vi "Meas_Fast_FID_Bkgnd.vi"(3 "Mode":T6, 5 "Traverse line In":T3 {"Carrier_2 Q (l/min)" format="%#.2f"; "Row Duration (mins)" format="%#.1f"; "Row No" min=0; "Trace Gas Concentration (%)" min=0.0 format="%#_4f"; "Carrier_1 Q (l/min)" format="%#.4f"; "Start X" format="%#.2f"; "Start Y" format="%#.2f"; "Start Z" format="%#.2f"; "End X" format="%#.2f"; "End Y" format="%#.2f"; "End Z" format="%#.2f"; "Tunnel Speed" format="%#.2f"; "Averaging time (mins)" min=0.0 format="%#.2f"}) -> (0 "Error Message":string, 1 "Status":T2, 2 "Traverse line Out":T3 {"Carrier_2 Q (l/min)" format="%#.2f"; "Row Duration (mins)" format="%#.1f"; "Row No" min=0; "Trace Gas Concentration (%)" min=0.0 format="%#_4f"; "Carrier_1 Q (l/min)" format="%#.4f"; "Start X" format="%#.2f"; "Start Y" format="%#.2f"; "Start Z" format="%#.2f"; "End X" format="%#.2f"; "End Y" format="%#.2f"; "End Z" format="%#.2f"; "Tunnel Speed" format="%#.2f"; "Averaging time (mins)" min=0.0 format="%#.2f"})   [LabVIEW 2022 SP3]
uses:
  Gen Trav/Traverse_cluster.ctl
  Gen Trav/Spacing.ctl
  Controls/Multi_run_mode.ctl
  Controls/User_Specific_mode.ctl
  Gen Trav/Multi_Run_Status.ctl
  FFID/Bkgnd Meas.ctl
  File/Setup_Filetype.ctl
  Gen Trav/Trav_mode.ctl
  Controls/Setup.ctl
  Controls/Save_Data.ctl
  Globals/Trav_pos_global.vi
  Globals/Extra_Commands_Global.vi
  Globals/Preference_global.vi
  Globals/Gas_management_global.vi
  Globals/Meas_global.vi
  <vilib>/Analysis/NI_AALPro.lvlib
  <vilib>/Analysis/NI_AALBase.lvlib
panel:
  out "Bkgnd Results":T1[][](array[typedef])
  in  "Cluster":T1
  out "C^2 too large":bool
  out "Block Number":i32
  out "Can Move Traverse?":bool
  out "Trace Q":dbl
  out "Trace on?":bool
  out "After First Move":sgl[][](array[numeric])
  out "Traverses":string[](array[string])
  out "Initial Trav Positions":sgl[][](array[numeric])
  out "First Bknd since calib":bool
  # "X           Y          Z"
  # "Start"
  # "End"
  # "X           Y          Z"
  # "Start"
  # "End"
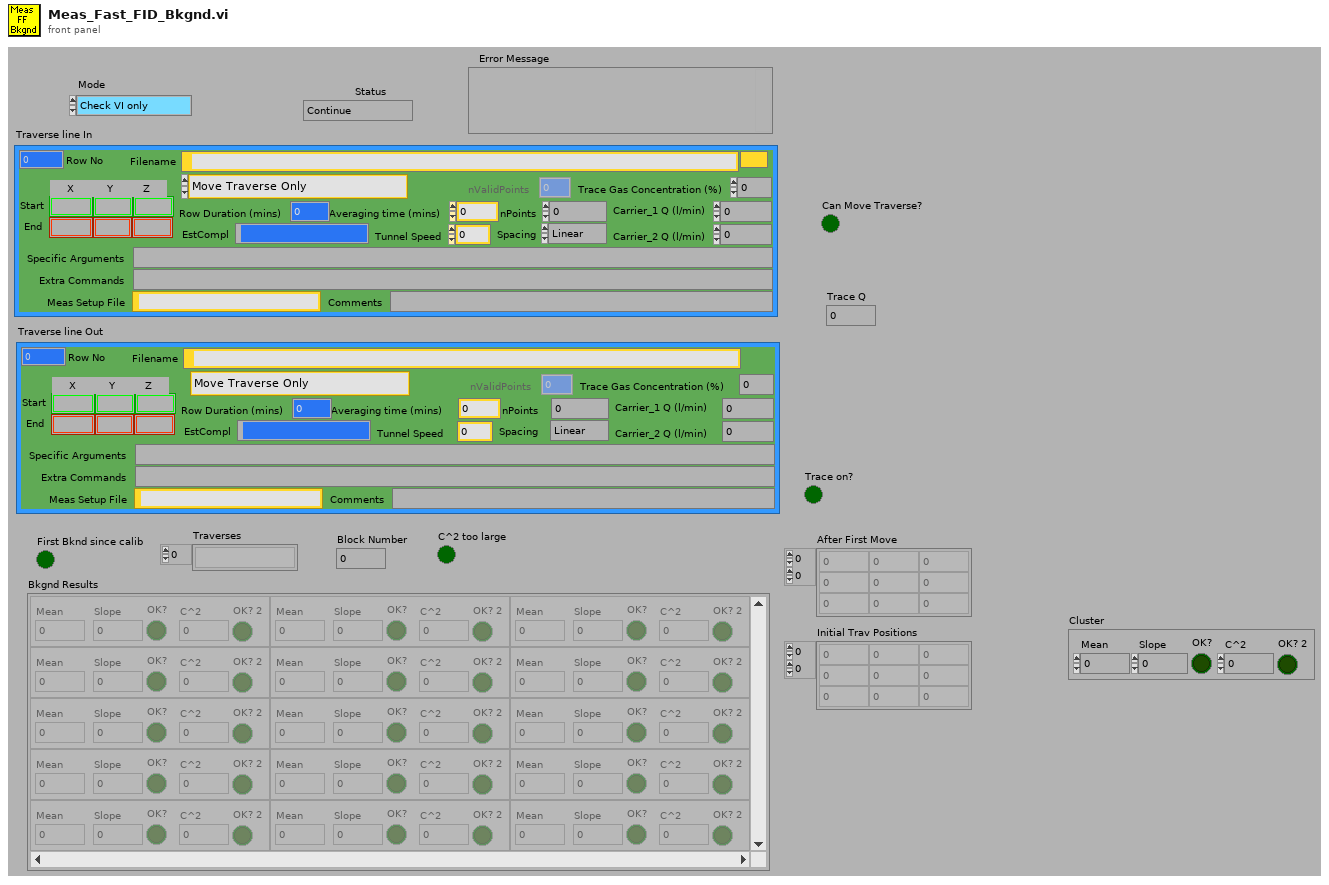
[diagram p1: front panel]
types:
  T1 = typedef "Bkgnd Meas.ctl" = cluster{"Mean":dbl, "Slope":dbl, "C^2":dbl, "OK?":bool, "OK? 2":bool}
  T2 = typedef "Multi_Run_Status.ctl" = enum16{"Continue", "Continue with Error", "Jump to Next Point", "Jump to Next Row", "Jump To Fall Back", "Terminate Run"}
  T3 = typedef "Traverse_cluster.ctl" = cluster{"Start X":sgl, "Start Y":sgl, "Start Z":sgl, "End X":sgl, "End Y":sgl, "End Z":sgl, "nPoints":i32, "Spacing":T4, "Filename":path, "Tunnel Speed":dbl, "Averaging time (mins)":dbl, "Extra Commands":string, "Carrier_1 Q (l/min)":dbl, "Carrier_2 Q (l/min)":dbl, "Trace Gas Concentration (%)":dbl, "Specific Arguments":string, "Comments":string, "Row No":i32, "Row Type Selector":T5, "EstCompl":string, "Row Duration (mins)":dbl, "nValidPoints":i32, "Meas Setup File":string}
  T4 = typedef "Spacing.ctl" = enum16{"Linear", "Log", "Gauss", "Specified", "N/A"}
  T5 = typedef "Multi_run_mode.ctl" = enum16{"Move Traverse Only", "Set Tunnel Speed Only", "Set Source Only", "Set Measurement Conditions", "Single Measurement", "Vertical Profile", "Lateral Profile", "Longitudinal Profile", "Multi-Axis Profile", "Explore Volume", "Auto Calibrate", "Meas Fast FID Bkgnd", "Check Beam Power", "Scanning Valve Measurement", "Run VI Named:", "Set ADAM Ch", "Wait (minutes)", "Send Message", "Synchronize With:", "Fall Back to this Row", "Turn Off Row Repeating", "Traverse 3D Volume", "Blank Row", "Jump to Fall Back Row"}
  T6 = typedef "User_Specific_mode.ctl" = enum16{"Check VI only", "Run VI"}
  T7 = typedef "Tunnel_Coordinates.ctl" = enum16{"Work in Tunnel Coordinates", "Work in Model Coordinates"}
  T8 = typedef "Setup_Filetype.ctl" = enum16{"Measurement Setups", "Calibration Setups", "General", "Results File Plotter Setups", "Speed Calib Tweaks"}
  T9 = typedef "Trav_mode.ctl" = enum16{"Move traverse", "Read traverse position", "Teach Position"}
  T10 = typedef "Save_Data.ctl" = enum16{"Save No Data", "Save Data"}
  T11 = typedef "Setup.ctl" = enum16{"Run Program", "Show Setup", "Save Current Setup", "Setup Front Panel"}
  T12 = typedef "GMU Gas Line Name.ctl" = enum16{"GMU1 Source", "GMU2 Source", "GMU2 Calib", "CPP GRC-A", "CPP GRC-B"}
  T13 = typedef "Analysis_info_cluster.ctl" = cluster{"Colour":u32, "Inst type":T14, "Inst name":string, "Symbol":string, "Code name":string, "Extra Info":string, "Inst Array":T15, "U":dbl, "u^2":dbl, "u^3":dbl, "u^4":dbl, "Skew_u":dbl, "Kurt_u":dbl, "Sd Error in Mean":dbl, "% u'/U":dbl, "X":dbl, "Y":dbl, "Z":dbl, "Timescale integral Estimate":dbl, "Sd Error in Variance":dbl, "Calib File":path, "Calib Constants":dbl[], "Output Position":bool, "Stats":enum16{"None", "Basic", "Full"}, "Av Sampling Rate":dbl, "Av No of Samples":dbl, "Total Meas Time (s)":dbl, "OrigChName":string, "Max value":dbl, "Min value":dbl, "Req Sample Rate Hz":dbl, "Sync Delay Time (s)":dbl, "Ch No":i16, "Device":string, "Use Latest Calib":bool, "Port":string, "Metadata Ch Names":string[], "Metadata Ch Values":string[], "Label":string, "chState":T16, "Point Drift":dbl, "inputConfig":string}
  T14 = typedef "Inst_type.ctl" = enum16{"Raw voltage", "Raw with zero offsetting", "Propeller anemometer", "Pressure Transducer", "Pitot-static tube", "Hot wire", "Cross wire 1", "Cross wire 2", "Generic Linear", "Generic Polynomial", "Generic BackPoly", "Fast FID", "Thermocouple", "Cold wire", "Pulsed Wire", "LDA Vel", "LDA Tran time", "LDA Arr time", "Microphone"}
  T15 = typedef "Instrument_Array.ctl" = enum16{"PWA", "LDA", "Analogue"}
  T16 = typedef "channelState.ctl" = enum32{"No Selection", "Solo", "Mute"}
  T17 = typedef "Time_Trace_Cluster.ctl" = cluster{"Weighting":dbl[], "Voltage":dbl[], "Eng Values":dbl[]}
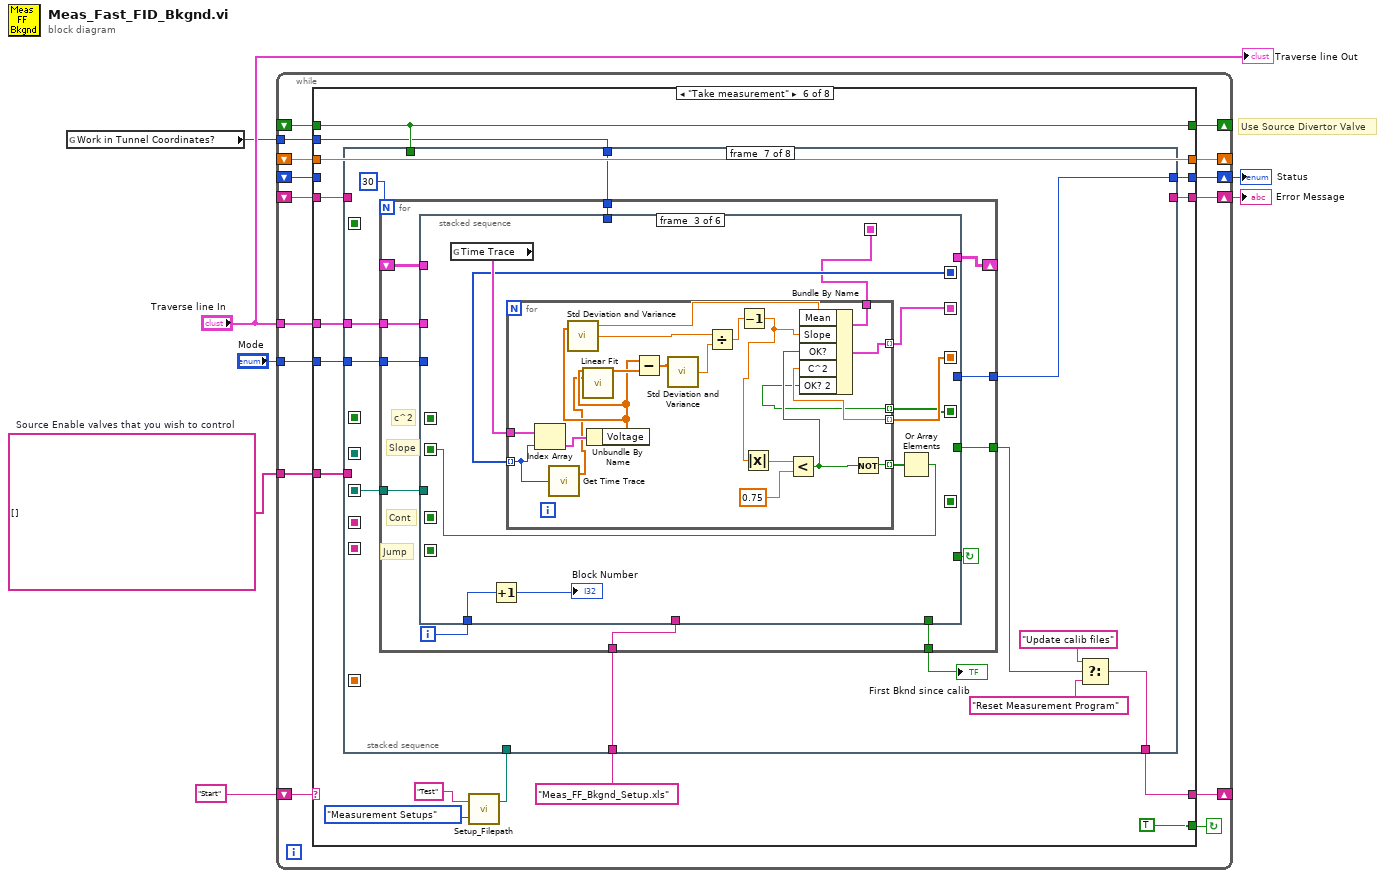
[diagram p0: block diagram]
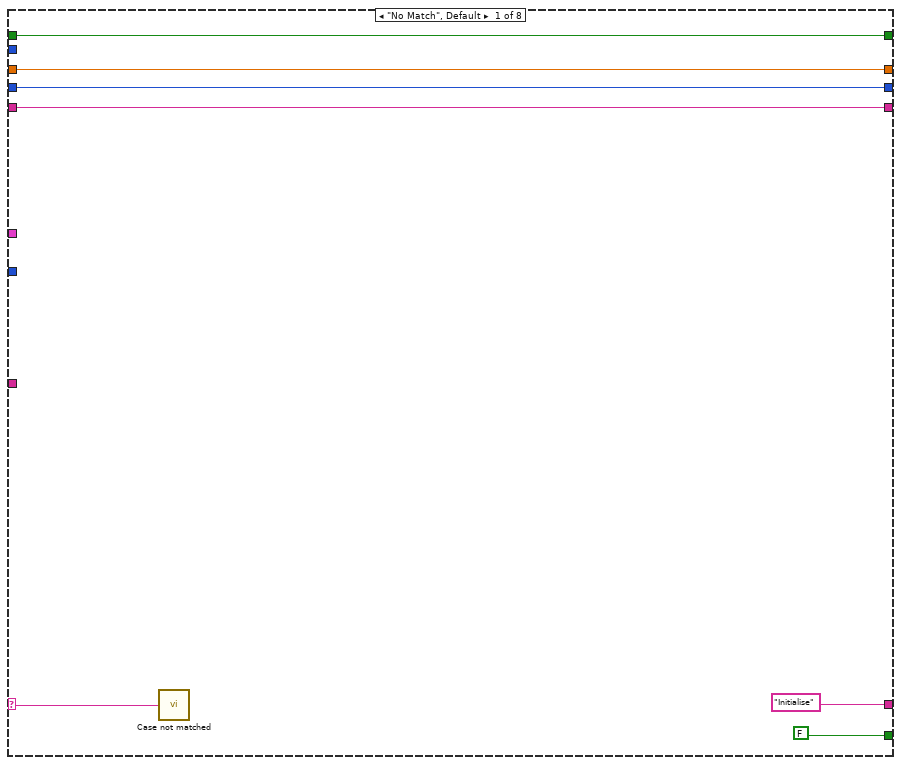
[diagram p2: hidden frame]
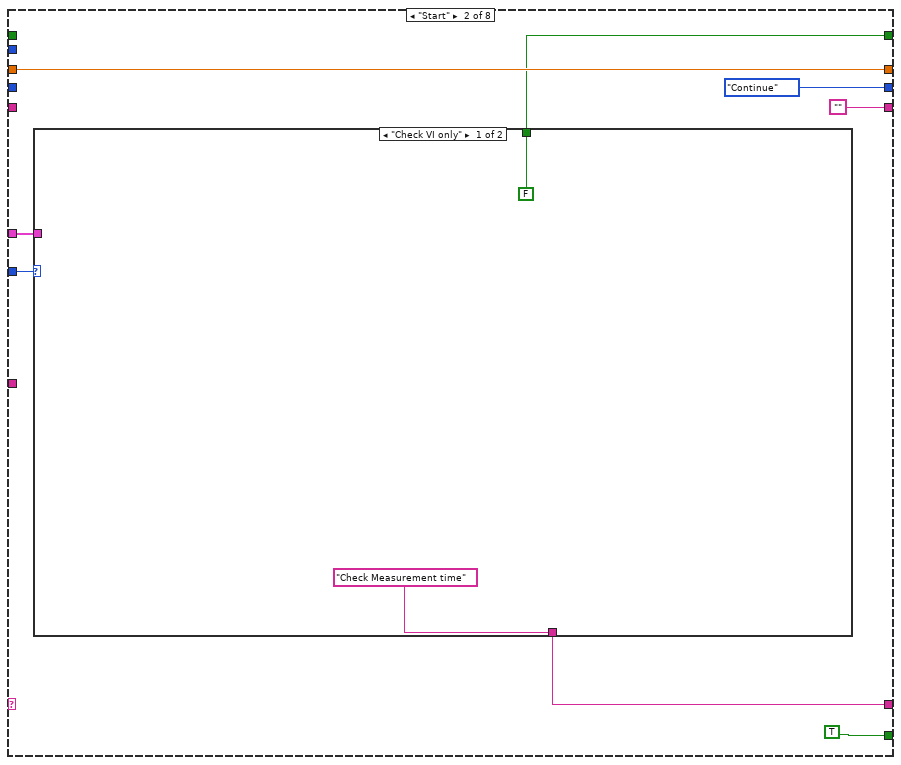
[diagram p3: hidden frame]
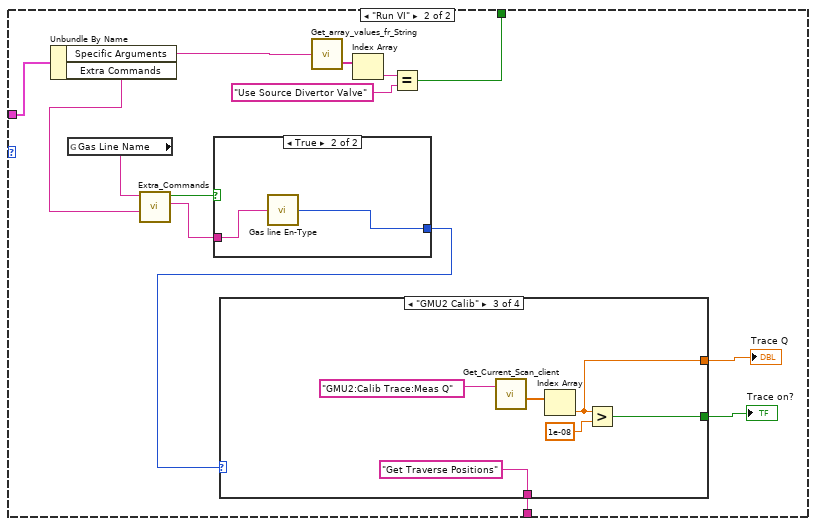
[diagram p4: hidden frame]
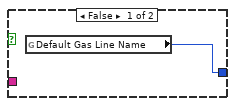
[diagram p5: hidden frame]
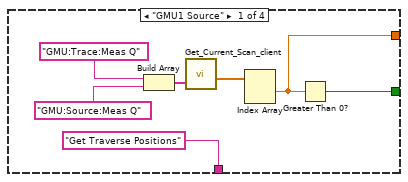
[diagram p6: hidden frame]
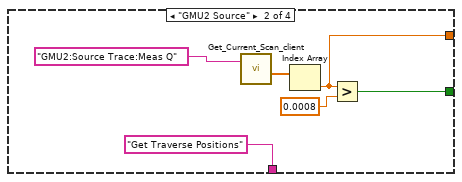
[diagram p7: hidden frame]
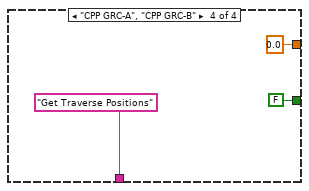
[diagram p8: hidden frame]
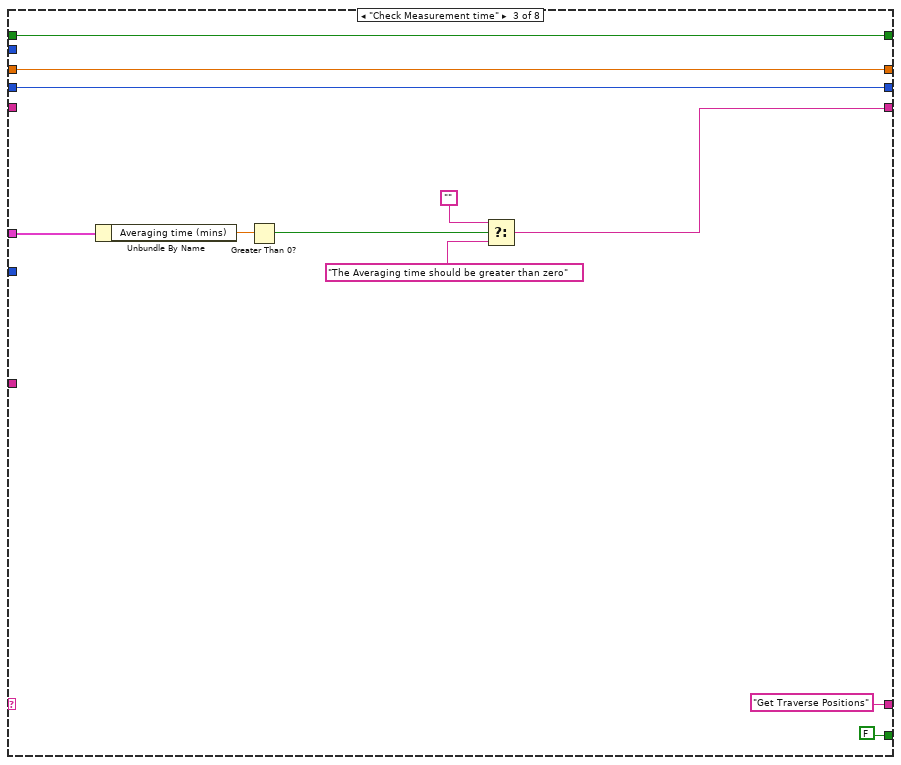
[diagram p9: hidden frame]
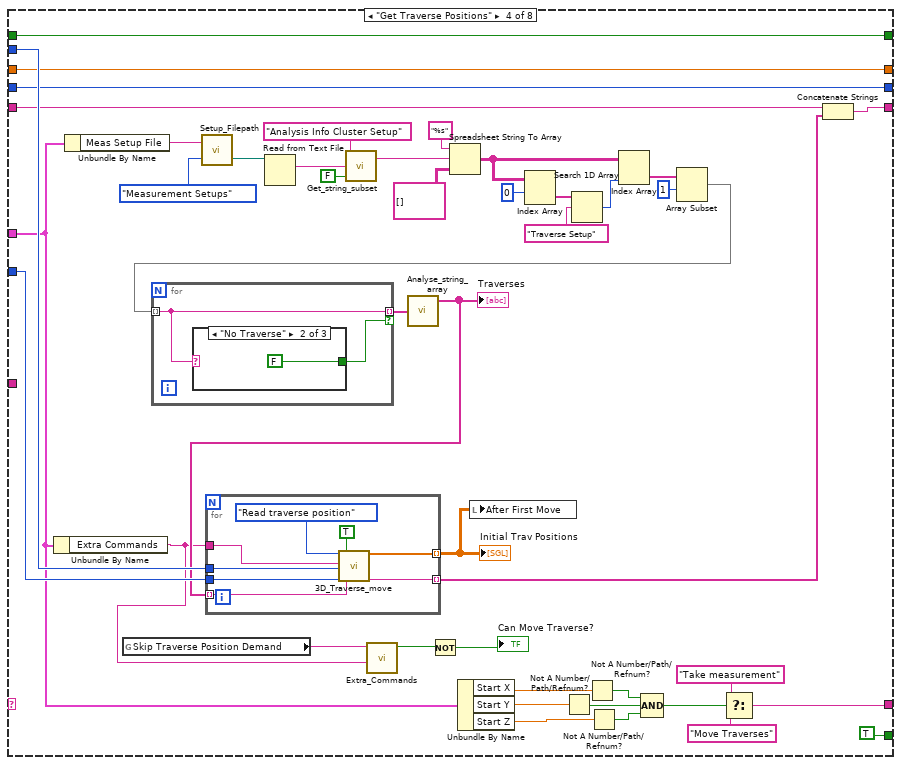
[diagram p10: hidden frame]
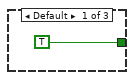
[diagram p11: hidden frame]
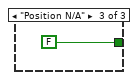
[diagram p12: hidden frame]
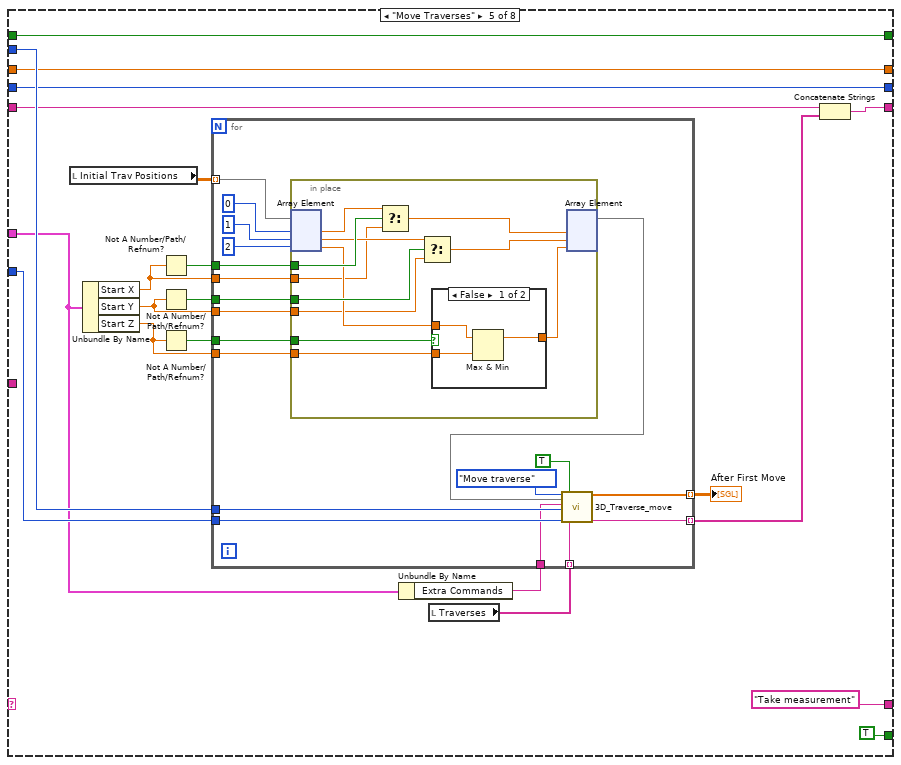
[diagram p13: hidden frame]
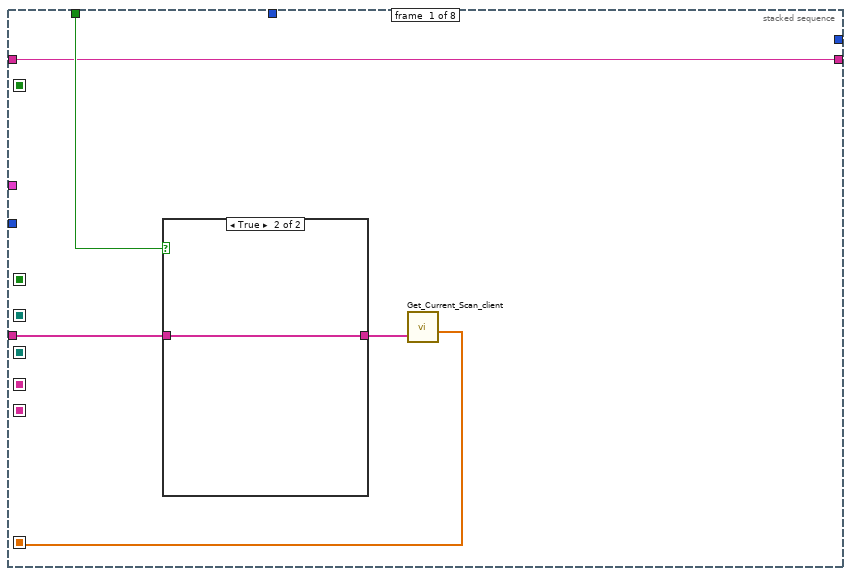
[diagram p15: hidden frame]
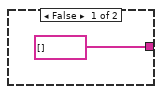
[diagram p16: hidden frame]
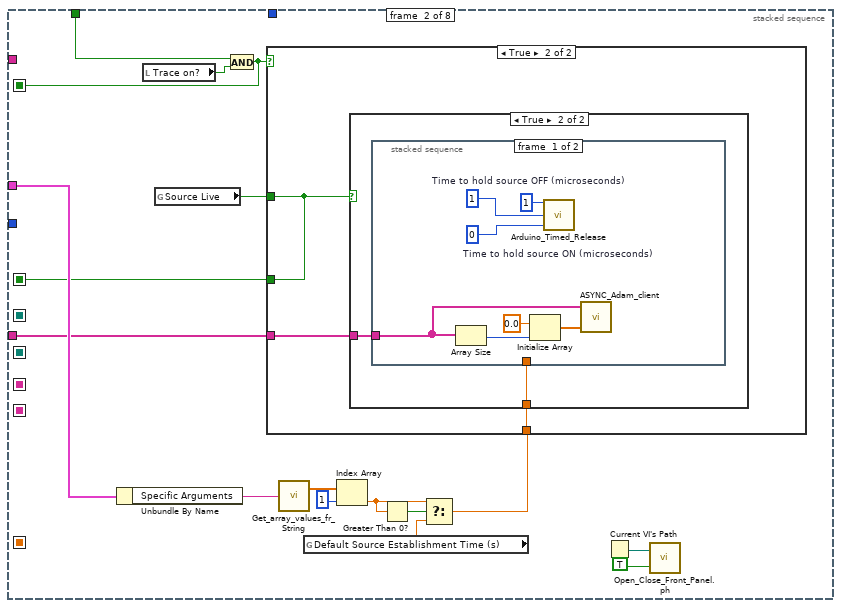
[diagram p17: hidden frame]
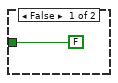
[diagram p18: hidden frame]
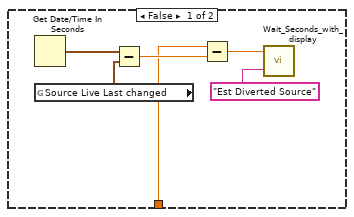
[diagram p19: hidden frame]
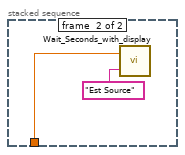
[diagram p20: hidden frame]
diagram:
  w1 = string[] []  # Source Enable valves that you wish to control
  # "Use Source Divertor Valve"
  n1 = global read "Trav_pos_global.vi" "Work in Tunnel Coordinates?"() -> (w2:T7)
  n2 = while {
    shift-left: "Start" -> [w20]
    shift-right: [w21] -> _
    shift-right: [w16] -> _
    shift-left: _ -> [w19]
    tunnel: "Mode" -> [w18]
    tunnel: "Traverse line In" -> [w17]
    shift-right: [w15] -> w5
    shift-left: _ -> [w13]
    shift-right: [w14] -> w3
    shift-left: _ -> [w12]
    tunnel: w2 -> [w11]
    shift-right: [w9] -> _
    shift-left: _ -> [w10]
    tunnel: w1 -> [w8]
    stop <- w22 continue-if-true
    n3 = case shown="\"Take measurement\"" w20 {
      selector: w20 -> [w23 _ _ _ _ _ _ _]
      tunnel: [FALSE TRUE FALSE TRUE TRUE TRUE TRUE FALSE] -> w22
      tunnel: ["Initialise" w35 "Get Traverse Positions" w120 "Take measurement" w212 "Reset Measurement Program" "End"] -> w21
      tunnel: w19 -> [w27 w33 w81 w127 w151 w216 w507 _]
      tunnel: w18 -> [_ w36 _ w129 w157 w207 _ _]
      tunnel: w17 -> [_ w30 w89 w95 w147 w215 _ _]
      tunnel: [w27 w33 w81 w127 w151 w216 w507 w512] -> w16
      tunnel: [w26 Multi_Run_Status."Continue" ("Status") w82 w126 w152 w213 w506 w511] -> w15
      tunnel: [w25 "" w85 w123 w154 w203 w505 w514] -> w14
      tunnel: w13 -> [w26 _ w82 w126 w152 _ w506 w511]
      tunnel: w12 -> [w25 _ _ w125 w155 w204 w505 w514]
      tunnel: w11 -> [_ _ _ w128 w156 w206 _ _]
      tunnel: w10 -> [w24 _ w80 w119 w167 w208 w502 w510]
      tunnel: [w24 w31 w80 w119 w167 w208 w502 w510] -> w9
      tunnel: w8 -> [_ _ _ _ _ w205 _ _]
      frame "No Match", Default {
        n4 = call "Case not matched.vi"("Case Name not Matched"=w23) -> ()
      }
      frame "Start" {
        n5 = case shown="\"Check VI only\"" w36 {
          tunnel: ["Check Measurement time" w45] -> w35
          tunnel: [FALSE w48] -> w31
          tunnel: w30 -> [_ w49]
          frame "Check VI only" {
          }
          frame "Run VI" {
            n6 = Unbundle By Name(w49) -> ("Specific Arguments"=w53:string, "Extra Commands"=w40:string)
            n7 = global read "Extra_Commands_Global.vi" "Gas Line Name"() -> (w44:string)
            n8 = call "Extra_Commands.vi"("String to Search"=w40, "Command"=w44) -> ("String Value"=w42:string, "Command Found"=w43:bool)  [unwired: 1 in, 3 out]
            n9 = case shown="True" w43 {
              tunnel: [w54 w55] -> w41
              tunnel: w42 -> [_ w56]
              frame False {
                n10 = global read "Trav_pos_global.vi" "Default Gas Line Name"() -> (w54:T12)
              }
              frame True {
                n11 = call "Gas line En-Type.vi"("Gas Line Name String"=w56) -> ("Gas Line Name"=w55:T12)  [unwired: 4 in]
              }
            }
            n12 = case shown="\"GMU2 Calib\"" w41 {
              tunnel: [w59 w66 w72 0.0] -> w47
              tunnel: [w58 w67 w73 FALSE] -> w46
              tunnel: ["Get Traverse Positions" "Get Traverse Positions" "Get Traverse Positions" "Get Traverse Positions"] -> w45
              frame "GMU1 Source" {
                n13 = Build Array("GMU:Trace:Meas Q", "GMU:Source:Meas Q") -> (w62:string[])
                n14 = call "Get_Current_Scan_client.vi"("multipleChannels"=w62) -> ("Numerical Values"=w60:dbl[])  [unwired: 1 in, 3 out]
                n15 = Index Array(array=w60) -> (element #1=w59:dbl)  [unwired: 2 in, 1 out]
                n16 = Greater Than 0?(x=w59) -> (x > 0?=w58:bool)
              }
              frame "GMU2 Source" {
                n17 = call "Get_Current_Scan_client.vi"("singleChannel"="GMU2:Source Trace:Meas Q") -> ("Numerical Values"=w69:dbl[])  [unwired: 1 in, 3 out]
                n18 = Index Array(array=w69) -> (element=w66:dbl)  [unwired: 1 in]
                n19 = Greater?(x=w66, y=0.0008) -> (0:w67:bool)
              }
              frame "GMU2 Calib" {
                n20 = call "Get_Current_Scan_client.vi"("singleChannel"="GMU2:Calib Trace:Meas Q") -> ("Numerical Values"=w75:dbl[])  [unwired: 1 in, 3 out]
                n21 = Index Array(array=w75) -> (element=w72:dbl)  [unwired: 1 in]
                n22 = Greater?(x=w72, y=1e-08) -> (0:w73:bool)
              }
              frame "CPP GRC-A", "CPP GRC-B" {
              }
            }
            "Trace on?" <- w46
            "Trace Q" <- w47
            n23 = call "Get_array_values_fr_String.vi"("String Value"=w53) -> ("String array"=w51:string[])  [unwired: 1 out]
            n24 = Index Array(array=w51) -> (element=w52:string)  [unwired: 1 in]
            n25 = Equal?(x=w52, y="Use Source Divertor Valve") -> (x = y?=w48:bool)
          }
        }
      }
      frame "Check Measurement time" {
        n26 = Unbundle By Name(w89) -> ("Averaging time (mins)"=w88:dbl)
        n27 = Greater Than 0?(x=w88) -> (x > 0?=w83:bool)
        n28 = Select(t="", s=w83, f="The Averaging time should be greater than zero") -> (s? t:f=w85:string)
      }
      frame "Get Traverse Positions" {
        n29 = Unbundle By Name(w95) -> ("Extra Commands"=w92:string)
        n30 = Unbundle By Name(w95) -> ("Meas Setup File"=w132:string)
        n31 = global read "Extra_Commands_Global.vi" "Skip Traverse Position Demand"() -> (w93:string)
        n32 = call "Setup_Filepath.vi"("Setup File Type"=Setup_Filetype."Measurement Setups", "Filename in"=w132) -> ("Filename Out"=w121:path)  [unwired: 1 out]
        n33 = Read from Text File(file (use dialog)=w121) -> (text=w130:string)  [unwired: 3 in, 3 out]
        n34 = call "Get_string_subset.vi"("Show Dialog?"=FALSE, "String to split"=w130, "File Label"="Analysis Info Cluster Setup" ("String Name")) -> ("Output string"=w107:string)  [unwired: 1 in, 1 out]
        n35 = call "Extra_Commands.vi"("String to Search"=w92, "Command"=w93) -> ("Command Found"=w91:bool)  [unwired: 1 in, 4 out]
        n36 = Not(x=w91) -> (.not. x?=→"Can Move Traverse?":bool)
        n37 = Spreadsheet String To Array(format string="%s", spreadsheet string=w107, array type (2D Dbl)=string[][] []) -> (array=w103:string[][])  [unwired: 1 in]
        n38 = Unbundle By Name(w95) -> ("Start X"=w118:sgl, "Start Y"=w117:sgl, "Start Z"=w116:sgl)
        n39 = Index Array(array=w103, index (row)=0) -> (element=w105:string[])  [unwired: 1 in]
        n40 = Not A Number/Path/Refnum?(number/path/refnum=w117) -> (NaN/Path/Refnum?=w114:bool)
        n41 = Search 1D Array(1D array=w105, element="Traverse Setup") -> (index of element=w102:i32)  [unwired: 1 out]
        n42 = Not A Number/Path/Refnum?(number/path/refnum=w118) -> (NaN/Path/Refnum?=w115:bool)
        n43 = Not A Number/Path/Refnum?(number/path/refnum=w116) -> (NaN/Path/Refnum?=w113:bool)
        n44 = Index Array(array=w103, index (col)=w102) -> (element=w101:string[])  [unwired: 1 in]
        n45 = Compound Arithmetic op=AND(w115, w114, w113) -> (w94:bool)
        n46 = Array Subset(array=w101, index=1) -> (w99:string[])  [unwired: 1 in]
        n47 = for {
          tunnel: [w142] -> w98 mode=indexing if=w143
          tunnel: w99 -> [w142] mode=indexing
          n48 = case shown="\"No Traverse\"" w142 {
            tunnel: [TRUE FALSE FALSE] -> w143
            frame Default {
            }
            frame "No Traverse" {
            }
            frame "Position N/A" {
            }
          }
        }
        n49 = call "Analyse_string_array.vi"("String array"=w98) -> ("Unique strings"=w97:string[])  [unwired: 1 in, 1 out]
        "Traverses" <- w97
        n50 = for {
          tunnel: w97 -> [w140] mode=indexing
          tunnel: w128 -> [w139]
          tunnel: w92 -> [w138]
          tunnel: w129 -> [w137]
          tunnel: [w136] -> w110 mode=indexing
          tunnel: [w135] -> w124 mode=indexing
          n51 = call "3D_Traverse_move.vi"("Mode"=Trav_mode."Read traverse position", "Extra command String"=w138, "Work in Tunnel Coordinates"=w139, "Simulate/Run"=w137, "Route Checking?"=TRUE, "Traverse name"=w140) -> ("Trav Position achieved"=w136:sgl[], "Error String"=w135:string)  [unwired: 10 in, 2 out]
        }
        "Initial Trav Positions" <- w110
        n52 = local write "After First Move"(w110) -> ()
        n53 = Select(t="Take measurement", s=w94, f="Move Traverses") -> (s? t:f=w120:string)
        n54 = Concatenate Strings(w125, w124) -> (w123:string)
      }
      frame "Move Traverses" {
        n55 = local read "Initial Trav Positions"() -> (w165:sgl[][])
        n56 = Unbundle By Name(w147) -> ("Start X"=w160:sgl, "Start Y"=w159:sgl, "Start Z"=w158:sgl)
        n57 = Not A Number/Path/Refnum?(number/path/refnum=w160) -> (NaN/Path/Refnum?=w163:bool)
        n58 = Not A Number/Path/Refnum?(number/path/refnum=w159) -> (NaN/Path/Refnum?=w162:bool)
        n59 = Not A Number/Path/Refnum?(number/path/refnum=w158) -> (NaN/Path/Refnum?=w161:bool)
        n60 = Unbundle By Name(w147) -> ("Extra Commands"=w164:string)
        n61 = local read "Traverses"() -> (w166:string[])
        n62 = for {
          tunnel: w166 -> [w186] mode=indexing
          tunnel: w157 -> [w185]
          tunnel: w156 -> [w184]
          tunnel: w165 -> [w181] mode=indexing
          tunnel: w164 -> [w182]
          tunnel: w163 -> [w180]
          tunnel: w162 -> [w179]
          tunnel: w161 -> [w178]
          tunnel: w160 -> [w177]
          tunnel: w159 -> [w176]
          tunnel: w158 -> [w175]
          tunnel: [w173] -> w153 mode=indexing
          tunnel: [w169] -> w148 mode=indexing
          n63 = in-place {
            in-place-border: w180 -> [w198]
            in-place-border: w179 -> [w197]
            in-place-border: w178 -> [w187]
            in-place-border: w177 -> [w190]
            in-place-border: w176 -> [w189]
            in-place-border: w175 -> [w188]
            n64 = in-place-array #1(w181, 0, 1, 2) -> (w196:sgl, w195:sgl, w194:sgl)
            n65 = Select(t=w196, s=w198, f=w190) -> (s? t:f=w193:sgl)
            n66 = Select(t=w195, s=w197, f=w189) -> (s? t:f=w192:sgl)
            n67 = case shown="False" w187 {
              tunnel: w194 -> [w200 w202]
              tunnel: [w199 w202] -> w191
              tunnel: w188 -> [w201 _]
              frame False {
                n68 = Max & Min(x=w200, y=w201) -> (max(x,y)=w199:sgl)  [unwired: 1 out]
              }
              frame True {
              }
            }
            n69 = in-place-array #1(w193, w192, w191) -> (w174:sgl[])  [unwired: 3 out]
          }
          n70 = call "3D_Traverse_move.vi"("Mode"=Trav_mode."Move traverse", "Position"=w174, "Extra command String"=w182, "Work in Tunnel Coordinates"=w184, "Simulate/Run"=w185, "Route Checking?"=TRUE, "Traverse name"=w186) -> ("Trav Position achieved"=w169:sgl[], "Error String"=w173:string)  [unwired: 9 in, 2 out]
        }
        "After First Move" <- w148
        n71 = Concatenate Strings(w155, w153) -> (w154:string)
      }
      frame "Take measurement" {
        n72 = call "Setup_Filepath.vi"("Setup File Type"=Setup_Filetype."Measurement Setups", "Filename in"="Test") -> ("Directory"=w209:path)  [unwired: 1 out]
        n73 = stacked-sequence {
          seq-local: [_ _ w271 _ _ _ _ _] -> [_ _ _ _ w288 _ _ _]
          seq-local: [_ _ _ _ w294 _ _ _] -> [_ _ _ _ _ w302 _ _]
          seq-local: [_ _ _ w275 _ _ _ _] -> [_ _ _ _ _ _ w320 _]
          seq-local: [_ _ _ w277 _ _ _ _] -> [_ _ _ _ w293 _ _ _]
          seq-local: [_ w230 _ _ _ _ _ _] -> [_ _ _ _ _ _ _ _]
          seq-local: [_ w225 _ _ _ _ _ _] -> [_ _ _ _ _ _ _ w482]
          seq-local: [w219 _ _ _ _ _ _ _] -> [_ _ _ _ _ _ _ w481]
          tunnel: "Meas_FF_Bkgnd_Setup.xls" -> [_ _ _ _ _ w304 w321 _]
          tunnel: w215 -> [_ w238 w268 _ w290 _ w313 w477]
          tunnel: [_ _ _ _ _ _ w319 _] -> w213
          tunnel: [_ _ _ _ _ _ w317 _] -> w212
          tunnel: w209 -> [_ _ w263 _ _ w300 _ _]
          tunnel: w208 -> [w222 w228 _ _ _ _ _ _]
          tunnel: w207 -> [_ _ _ _ _ _ w311 w478]
          tunnel: w206 -> [_ _ _ _ _ _ w312 w479]
          tunnel: w205 -> [w221 w229 _ _ _ _ _ w480]
          tunnel: w204 -> [w218 _ _ _ _ _ _ _]
          tunnel: [w218 _ _ _ _ _ _ _] -> w203
          frame #0 {
            n74 = case shown="True" w222 {
              tunnel: w221 -> [_ w224]
              tunnel: [string[] [] ("appended array") w224] -> w220
              frame False {
              }
              frame True {
              }
            }
            n75 = call "Get_Current_Scan_client.vi"("multipleChannels"=w220) -> ("Numerical Values"=w219:dbl[])  [unwired: 1 in, 3 out]
          }
          frame #1 {
            n76 = Unbundle By Name(w238) -> ("Specific Arguments"=w237:string)
            n77 = local read "Trace on?"() -> (w227:bool)
            n78 = global read "Gas_management_global.vi" "Source Live"() -> (w226:bool)
            n79 = And(x=w228, y=w227) -> (x .and. y?=w230:bool)
            n80 = call "Get_array_values_fr_String.vi"("String Value"=w237) -> ("Numeric Array"=w235:dbl[])  [unwired: 1 out]
            n81 = global read "Preference_global.vi" "Default Source Establishment Time (s)"() -> (w232:dbl)
            n82 = Index Array(array=w235, index=1) -> (element=w233:dbl)
            n83 = Greater Than 0?(x=w233) -> (x > 0?=w234:bool)
            n84 = Select(t=w233, s=w234, f=w232) -> (s? t:f=w231:dbl)
            n85 = case shown="True" w230 {
              tunnel: w231 -> [_ w244]
              tunnel: [FALSE w242] -> w225
              tunnel: w229 -> [_ w243]
              tunnel: w226 -> [_ w242]
              frame False {
              }
              frame True {
                n86 = case shown="True" w242 {
                  tunnel: w244 -> [w245 w252]
                  tunnel: w243 -> [_ w251]
                  frame False {
                    n87 = Get Date/Time In Seconds() -> (seconds since 1Jan1904=w246:timestamp)
                    n88 = global read "Gas_management_global.vi" "Source Live Last changed"() -> (w247:timestamp)
                    n89 = Subtract(x=w246, y=w247) -> (x-y=w248:dbl)
                    n90 = Subtract(x=w245, y=w248) -> (x-y=w250:dbl)
                    n91 = call "Wait_Seconds_with_display.vi"("Message"="Est Diverted Source", "Seconds to wait"=w250) -> ()  [unwired: 2 out]
                  }
                  frame True {
                    n92 = stacked-sequence {
                      tunnel: w252 -> [_ w260]
                      tunnel: w251 -> [w256 _]
                      frame #0 {
                        w257 = u32 1  # Time to hold source OFF (microseconds)
                        w258 = u32 0  # Time to hold source ON (microseconds)
                        n93 = Array Size(array=w256) -> (size(s)=w255:i32)
                        n94 = Initialize Array(0.0 ("element"), w255) -> (w253:dbl[])
                        n95 = call "Arduino_Timed_Release.vi"("Time to hold source ON (microseconds)"=w258, "Time to hold source OFF (microseconds)"=w257, "Number of cycles"=u16 1) -> ()  [unwired: 2 out]
                        n96 = call "ASYNC_Adam_client.vi"("Values"=w253, "Channel Names"=w256) -> ()  [unwired: 1 in, 2 out]
                      }
                      frame #1 {
                        n97 = call "Wait_Seconds_with_display.vi"("Message"="Est Source", "Seconds to wait"=w260) -> ()  [unwired: 2 out]
                      }
                    }
                  }
                }
              }
            }
            n98 = Current VI's Path() -> (path=w239:path)
            n99 = call "Open_Close_Front_Panel.ph.vi"("openWindow (T)"=TRUE ("Front Panel Window:Open"), "VI path"=w239) -> ()  [unwired: 1 in, 1 out]
          }
          frame #2 {
            w269 = TRUE  # Show Dialog?
            n100 = Unbundle By Name(w268) -> ("Meas Setup File"=w266:string)
            n101 = Match Pattern(string=w266, regular expression=";") -> (before substring=w265:string)  [unwired: 4 out]
            n102 = Build Path(base path=w263, name or relative path=w265) -> (appended path=w270:path)
            n103 = Format Into String(format string="Meas Setup File   %s", w263) -> (resulting string=w262:string)  [unwired: 2 in, 1 out]
            n104 = call "Read_spec_No_of_Characters.vi"("Filename"=w270) -> ("character string"=w272:string)  [unwired: 1 out]
            n105 = call "Get_string_subset.vi"("String Name"=w262, "Show Dialog?"=w269, "String to split"=w272, "File Label"="Raw data header") -> ("Output string"=w271:string)  [unwired: 1 out]
          }
          frame #3 {
            n106 = call "Create_Error_log_folders.vi"("Log Filename"="FF_Bkgnd_Info.xls") -> ("Local Log File"=w277:path)  [unwired: 5 in, 1 out]
            n107 = call "Get_Data_Base_file_code.vi"("Data Type"="Raw_Calibrations", "Results Filename"=w277, "Short_Name"="Raw_Cal") -> ("Raw Data File Name"=w275:path)  [unwired: 1 in, 3 out]
          }
          frame #4 {
            n108 = Unbundle By Name(w290) -> ("Averaging time (mins)"=w289:dbl)
            n109 = Path To String(path=w293) -> (string=w292:string)
            n110 = Multiply(x=w289, y=60.0) -> (x*y=w286:dbl)
            n111 = Number To Decimal String(number=w286) -> (decimal integer string=w299:string)  [unwired: 1 out]
            n112 = call "Replace_data_in_setup_string.vi"("New data string"=w299, "Input string"=w288, "Variable name"="Time per Block (s)") -> ("Appended string"=w284:string)
            n113 = call "Replace_data_in_setup_string.vi"("New data string"="", "Input string"=w284, "Variable name"="Per Block_Plug_Ins") -> ("Appended string"=w281:string)
            n114 = call "Replace_data_in_setup_string.vi"("New data string"="1", "Input string"=w281, "Variable name"="No of blocks") -> ("Appended string"=w280:string)
            n115 = call "Replace_data_in_setup_string.vi"("New data string"="No LDA data", "Input string"=w280, "Variable name"="LDA data" ("Label for characters")) -> ("Appended string"=w295:string)
            n116 = call "Replace_data_in_setup_string.vi"("New data string"=w292, "Input string"=w295, "Variable name"="Results filename") -> ("Appended string"=w294:string)
          }
          frame #5 {
            w308 = FALSE  # advisory dialog? (display:T)
            w309 = FALSE  # append to file? (new file:F)
            n117 = call "Remove_Plug_Ins_etc.vi"("Input String"=w302) -> ("Output string"=w301:string)
            n118 = call "Add_label_to_string.vi"("String to write"=w301, "File Label"="Raw data header") -> ("Output string"=w305:string)
            n119 = Build Path(base path=w300, name or relative path=w304) -> (appended path=w303:path)
            n120 = call "Add_length_to_string.vi"("String in"=w305) -> ("String out"=w307:string)
            n121 = call "Write_Characters_To_File.vi"("file path (dialog if empty)"=w303, "advisory dialog? (display:T)"=w308, "character string"=w307, "append to file? (new file:F)"=w309) -> ()  [unwired: 1 in, 4 out]
          }
          frame #6 {
            n122 = for {
              N: 30 -> [_]
              tunnel: w321 -> [w333]
              tunnel: w320 -> [w332]
              tunnel: [w331] -> w319
              tunnel: [w330] -> w318
              tunnel: w313 -> [w328]
              tunnel: w312 -> [w327]
              tunnel: w311 -> [w326]
              tunnel: [w324] -> w310
              shift-right: [w322] -> _
              shift-left: _ -> [w323]
              i -> [w325]
              stop <- w329 continue-if-true
              # "Jump"
              # "Cont"
              # "Slope"
              # "c^2"
              n123 = stacked-sequence {
                seq-local: [w337 _ _ _ _ _] -> [_ _ _ w412 _ _]
                seq-local: [_ _ _ w415 _ _] -> [_ _ _ _ w432 _]
                seq-local: [_ w353 _ _ _ _] -> [_ _ _ w411 _ _]
                seq-local: [_ w349 _ _ _ _] -> [_ _ w389 _ _ _]
                seq-local: [_ _ w387 _ _ _] -> [_ _ _ w413 _ _]
                seq-local: [_ _ _ w414 _ _] -> [_ _ _ _ w431 _]
                seq-local: ["Cluster" _ _ _ _ _] -> [_ _ w384 _ _ _]
                seq-local: [_ w346 _ _ _ _] -> [_ _ w382 _ _ _]
                seq-local: [_ w347 _ _ _ _] -> [_ _ w383 _ _ _]
                seq-local: [_ _ w381 _ _ _] -> [_ _ _ _ _ w468]
                tunnel: w333 -> [w343 _ _ _ _ _]
                tunnel: w332 -> [w341 _ _ _ _ _]
                tunnel: [w339 _ _ _ _ _] -> w331
                tunnel: [w337 _ _ _ _ _] -> w330
                tunnel: [_ _ _ _ w430 _] -> w329
                tunnel: w328 -> [w335 _ _ _ w436 _]
                tunnel: w327 -> [_ _ _ _ w435 _]
                tunnel: w326 -> [_ _ _ _ w434 _]
                tunnel: w325 -> [_ _ w386 _ w433 w470]
                tunnel: [_ w348 _ _ _ _] -> w324
                tunnel: w323 -> [_ _ _ _ _ w469]
                tunnel: [_ _ _ _ _ w467] -> w322
                frame #0 {
                  w345 = TRUE  # Remote control
                  n124 = Unbundle By Name(w335) -> ("Extra Commands"=w336:string)
                  n125 = call "Code_to_run.vi"("Extra command String"=w336, "Raw data option"=enum16{"Save raw data", "Raw data not saved"}."Save raw data", "setup"=Setup."Run Program", "Remote control"=w345, "File"=Save_Data."Save Data", "Raw data file"=w341, "Setup filename"=w343) -> ("Status"=w339:T2)  [unwired: 5 in, 3 out]
                  n126 = Equal?(x=w339, y=Multi_Run_Status."Continue" ("Status")) -> (x = y?=w337:bool)
                }
                frame #1 {
                  n127 = global read "Meas_global.vi" "Analysis Info cluster"() -> (w350:T13[])
                  n128 = for {
                    tunnel: [w360] -> w352 mode=indexing
                    tunnel: [w359] -> w351 mode=indexing
                    tunnel: w350 -> [w358] mode=indexing
                    tunnel: [w357] -> w349 mode=indexing if=w354
                    tunnel: [w356] -> w347 mode=indexing if=w354
                    tunnel: [w355] -> w346 mode=indexing if=w354
                    i -> [w357]
                    n129 = Unbundle By Name(w358) -> ("Inst type"=w361:T14)
                    n130 = case shown="\"Fast FID\"" w361 {
                      tunnel: w358 -> [_ w380]
                      tunnel: [w364 w366] -> w360
                      tunnel: [FALSE w373] -> w359
                      tunnel: [w364 TRUE] -> w354
                      tunnel: [0.0 ("u^2") w368] -> w356
                      tunnel: [FALSE w367] -> w355
                      frame Default {
                        w364 = FALSE
                      }
                      frame "Fast FID" {
                        n131 = Unbundle By Name(w380) -> ("u^2"=w368:dbl, "Calib Constants"=w376:dbl[])
                        n132 = Index Array(array=w376, index=4) -> (element=w375:dbl)
                        n133 = Index Array(array=w376, index=3 ("Index")) -> (element=w378:dbl)
                        n134 = Multiply(x=w375, y=5.0) -> (x*y=w370:dbl)
                        n135 = Equal To 0?(x=w378) -> (x = 0?=w373:bool)
                        n136 = Max & Min(x=w370, y=0.3) -> (max(x,y)=w369:dbl)  [unwired: 1 out]
                        n137 = Greater?(x=w368, y=w369) -> (0:w366:bool)
                        n138 = Not(x=w366) -> (.not. x?=w367:bool)
                      }
                    }
                  }
                  n139 = Or Array Elements(Boolean array=w351) -> (logical OR=w348:bool)
                  n140 = Or Array Elements(Boolean array=w352) -> (logical OR=w353:bool)
                  "C^2 too large" <- w353
                }
                frame #2 {
                  n141 = global read "Meas_global.vi" "Time Trace"() -> (w390:T17[])
                  n142 = Increment(x=w386) -> (x+1=→"Block Number":i32)
                  n143 = for {
                    tunnel: w389 -> [w408] mode=indexing
                    tunnel: w390 -> [w410]
                    tunnel: [w398] -> w388 mode=indexing
                    tunnel: w384 -> [w407]
                    tunnel: [w406] -> w381 mode=indexing
                    tunnel: w383 -> [w394] mode=indexing
                    tunnel: w382 -> [w393] mode=indexing
                    n144 = Index Array(array=w410, index=w408) -> (element=w409:T17)
                    n145 = call "Get Time Trace.vi"("Channel Index"=w408) -> ("Time (s)"=w400:dbl[])  [unwired: 1 out]
                    n146 = Unbundle By Name(w409) -> ("Voltage"=w401:dbl[])
                    n147 = call <vilib>:"Std Deviation and Variance.vi"("X"=w401) -> ("mean"=w391:dbl, "standard deviation"=w404:dbl)  [unwired: 1 in, 1 out]
                    n148 = call <vilib>:"Linear Fit.vi"("Y"=w401, "X"=w400) -> ("Best Linear Fit"=w402:dbl[])  [unwired: 9 in, 4 out]
                    n149 = Subtract(x=w401, y=w402) -> (x-y=w403:dbl[])
                    n150 = call <vilib>:"Std Deviation and Variance.vi"("X"=w403) -> ("standard deviation"=w405:dbl)  [unwired: 1 in, 2 out]
                    n151 = Divide(x=w404, y=w405) -> (x/y=w399:dbl)
                    n152 = Decrement(x=w399) -> (x-1=w392:dbl)
                    n153 = Absolute Value(x=w392) -> (abs(x)=w396:dbl)
                    n154 = Less?(x=w396, y=0.75) -> (x < y?=w395:bool)
                    n155 = Bundle By Name(cluster=w407, "Mean"=w391, "Slope"=w392, "OK?"=w395, "C^2"=w394, "OK? 2"=w393) -> (w406:T1)
                    n156 = Not(x=w395) -> (.not. x?=w398:bool)
                  }
                  n157 = Or Array Elements(Boolean array=w388) -> (logical OR=w387:bool)
                }
                frame #3 {
                  n158 = case shown="False" w412 {
                    tunnel: [FALSE ("Can Move Traverse?") w421] -> w415
                    tunnel: [FALSE w420] -> w414
                    tunnel: w413 -> [_ w419]
                    tunnel: w411 -> [_ w418]
                    frame False {
                    }
                    frame True {
                      n159 = case shown="True" w419 {
                        tunnel: [w423 TRUE] -> w420
                        tunnel: [w424 w429] -> w421
                        tunnel: w418 -> [w422 _]
                        frame False {
                          n160 = case shown="True" w422 {
                            tunnel: [w425 w427] -> w424
                            tunnel: [w425 TRUE] -> w423
                            frame False {
                              w425 = FALSE ("Can Move Traverse?")
                            }
                            frame True {
                              n161 = local read "Can Move Traverse?"() -> (w427:bool)
                            }
                          }
                        }
                        frame True {
                          n162 = local read "Can Move Traverse?"() -> (w429:bool)
                        }
                      }
                    }
                  }
                }
                frame #4 {
                  n163 = case shown="True" w432 {
                    tunnel: w436 -> [_ w444]
                    tunnel: w435 -> [_ w447]
                    tunnel: w434 -> [_ w446]
                    tunnel: w433 -> [_ w450]
                    tunnel: w431 -> [w437 w439]
                    tunnel: [w437 w438] -> w430
                    frame False {
                    }
                    frame True {
                      n164 = local read "After First Move"() -> (w448:sgl[][])
                      n165 = Increment(x=w450) -> (x+1=w449:i32)
                      n166 = Unbundle By Name(w444) -> ("Extra Commands"=w443:string)
                      n167 = local read "Traverses"() -> (w445:string[])
                      n168 = for {
                        tunnel: w449 -> [w462]
                        tunnel: w448 -> [w459] mode=indexing
                        tunnel: w447 -> [w457]
                        tunnel: w446 -> [w456]
                        tunnel: w445 -> [w455] mode=indexing
                        tunnel: w443 -> [w454]
                        tunnel: Trav_mode."Move traverse" ("Mode") -> [w452]
                        tunnel: [w451] -> w441 mode=concatenating
                        n169 = Multiply(x=w462, y=sgl 100.0) -> (x*y=w460:sgl)
                        n170 = in-place {
                          in-place-border: w460 -> [w465]
                          n171 = in-place-array #2(w459, 2) -> (w466:sgl)
                          n172 = Add(x=w466, y=w465) -> (x+y=w464:sgl)
                          n173 = in-place-array #2(w464) -> (w458:sgl[])  [unwired: 1 out]
                        }
                        n174 = call "3D_Traverse_move.vi"("Mode"=w452, "Position"=w458, "Extra command String"=w454, "Work in Tunnel Coordinates"=w457, "Simulate/Run"=w456, "Route Checking?"=TRUE, "Traverse name"=w455) -> ("Error String"=w451:string)  [unwired: 9 in, 3 out]
                      }
                      n175 = Empty String/Path?(string/path=w441) -> (empty?=w440:bool)
                      n176 = And(x=w439, y=w440) -> (x .and. y?=w438:bool)
                    }
                  }
                }
                frame #5 {
                  n177 = case shown="1, Default" w470 {
                    tunnel: w468 -> [w472 w474]
                    tunnel: [w471 w473] -> w467
                    tunnel: w469 -> [_ w475]
                    frame 0 {
                      n178 = Build Array(w472) -> (w471:T1[][])
                    }
                    frame 1, Default {
                      n179 = Build Array (concatenate)(w475, w474) -> (w473:T1[][])
                    }
                  }
                  "Bkgnd Results" <- w467
                }
              }
            }
            "First Bknd since calib" <- w310
            n180 = Select(t="Update calib files", s=w318, f="Reset Measurement Program") -> (s? t:f=w317:string)
          }
          frame #7 {
            n181 = local read "Can Move Traverse?"() -> (w476:bool)
            n182 = case shown="True" w482 {
              tunnel: w481 -> [_ w497]
              tunnel: w480 -> [_ w496]
              frame False {
              }
              frame True {
                w498 = u32 0  # Time to hold source OFF (microseconds)
                w499 = u32 1  # Time to hold source ON (microseconds)
                n183 = call "ASYNC_Adam_client.vi"("Values"=w497, "Channel Names"=w496) -> ()  [unwired: 1 in, 2 out]
                n184 = call "Arduino_Timed_Release.vi"("Time to hold source ON (microseconds)"=w499, "Time to hold source OFF (microseconds)"=w498, "Number of cycles"=u16 1) -> ()  [unwired: 2 out]
              }
            }
            n185 = case shown="True" w476 {
              tunnel: w479 -> [_ w485]
              tunnel: w478 -> [_ w484]
              tunnel: w477 -> [_ w483]
              frame False {
              }
              frame True {
                n186 = local read "Initial Trav Positions"() -> (w487:sgl[][])
                n187 = Unbundle By Name(w483) -> ("Extra Commands"=w486:string)
                n188 = local read "Traverses"() -> (w488:string[])
                n189 = for {
                  tunnel: w488 -> [w495] mode=indexing
                  tunnel: w484 -> [w494]
                  tunnel: w485 -> [w493]
                  tunnel: w487 -> [w491] mode=indexing
                  tunnel: w486 -> [w490]
                  n190 = call "3D_Traverse_move.vi"("Mode"=Trav_mode."Move traverse", "Position"=w491, "Extra command String"=w490, "Work in Tunnel Coordinates"=w493, "Simulate/Run"=w494, "Route Checking?"=TRUE, "Traverse name"=w495) -> ()  [unwired: 9 in, 4 out]
                }
              }
            }
          }
        }
      }
      frame "Update calib files" {
        w503 = dbl[] [] ("C (ppm)")
        w504 = TRUE  # Specific Bkgnd Meas?
        n191 = local read "First Bknd since calib"() -> (w501:bool)
        n192 = call "Update_FFID_Bkgnd_info.vi"("First Bknd since calib"=w501, "c^2 (ppm^2)"=w503, "Specific Bkgnd Meas?"=w504, "C (ppm)"=w503) -> ()  [unwired: 1 in]
      }
      frame "Reset Measurement Program" {
        n193 = Get Date/Time In Seconds() -> (seconds since 1Jan1904=w513:timestamp)
        n194 = To Double Precision Float(number=w513) -> (double precision float=w512:dbl)
      }
    }
  }
  "Error Message" <- w3
  "Status" <- w5
  "Traverse line Out" <- "Traverse line In"
